vi "Check Grabs Done.vi"(8 "Increment?":bool, 9 "Grabs Finished":u16, 11 "Grabs to Acquire":u16) -> (0 "Next Grab Last":bool, 1 "Updated Grabs Finished":u16, 2 "Is NumGrabs >0?":bool, 3 "Grabs Done?":bool)   [LabVIEW 2014]
panel:
  # "Copyright 2014 Vidrio Technologies\nScanImage 5 software is licensed under the Apache License, Version 2.0 (the \"License\"); you may not use any files contained\nwithin the ScanImage 5 release except in compliance with the License. You may obtain a copy of the License at\n http://www.apache.org/licenses/LICENSE-2.0\nUnless required by applicable law or agreed to in writing, software distributed under the License is distributed on an\n\"AS IS\" BASIS, WITHOUT WARRANTIES OR CONDITIONS OF ANY KIND, either express or implied. See the License for the\n specific language governing permissions and limitations under the License."
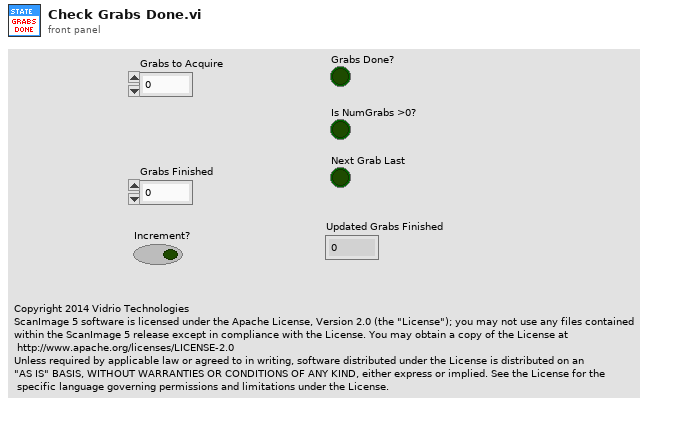
[diagram p1: front panel]
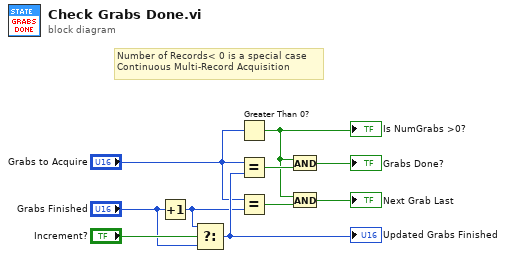
[diagram p0: block diagram]
diagram:
  # "Number of Records< 0 is a special case\nContinuous Multi-Record Acquisition"
  n1 = Increment(x="Grabs Finished") -> (x+1=w5:u16)
  n2 = Select(t=w5, s="Increment?", f="Grabs Finished") -> (s? t:f=w8:u16)
  "Updated Grabs Finished" <- w8
  n3 = Greater Than 0?(x="Grabs to Acquire") -> (x > 0?=w2:bool)
  "Is NumGrabs >0?" <- w2
  n4 = Equal?(x="Grabs to Acquire", y=w8) -> (x = y?=w7:bool)
  n5 = Equal?(x="Grabs to Acquire", y=w5) -> (x = y?=w3:bool)
  n6 = And(x=w2, y=w7) -> (x .and. y?=→"Grabs Done?":bool)
  n7 = And(x=w2, y=w3) -> (x .and. y?=→"Next Grab Last":bool)
